vi "GlobalACT.vi"() -> ()   [LabVIEW 2010]
panel:
  in  "Act Command":cluster{"Velocity":dbl, "Direction":dbl}
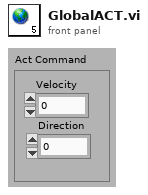
[diagram p1: front panel]
diagram:
